vi "Read Functions.vi"(9 "PythonConverter_BD in":refnum<class "PyConvBD.lvclass">) -> (3 "PythonConverter_BD out":refnum<class "PyConvBD.lvclass">, 4 "Functions":variant)   [LabVIEW 2014, in "PyConvBD.lvclass"]
uses:
  PyConvBD.lvclass
  PyConvBD.lvclass/PyConvBD.ctl
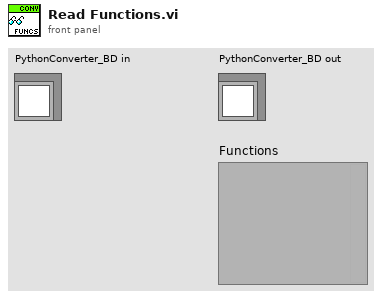
[diagram p1: front panel]
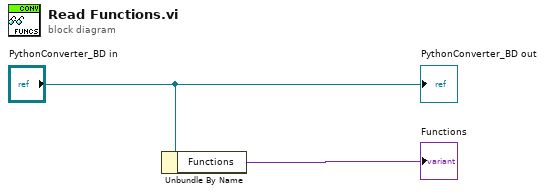
[diagram p0: block diagram]
diagram:
  n1 = Unbundle By Name("PythonConverter_BD in") -> ("Functions"=→"Functions":variant)
  "PythonConverter_BD out" <- "PythonConverter_BD in"
